vi "Begin.vi"(11 "Image Size":T1=enum."160x120") -> ()   [LabVIEW 2012]
doc: "Called before other user functions, this VI is expected to open initial I/O refnums, load in file data, and do all program initialization. Notice that the <B>error out</B> terminal is simply used for data flow. Wiring it to other structures or subVIs ensures that this VI runs first."
uses:
  <vilib>/Rock Robotics/WPI/Camera/WPI_CameraImageSize.ctl
  <vilib>/Rock Robotics/WPI/DriverStation/WPI_DriverStationRobotMode2.ctl
  <vilib>/Rock Robotics/WPI/Joystick/WPI_JoystickDeviceEnum.ctl
  <vilib>/Rock Robotics/WPI/CAN/Jaguar/SubVIs/WPI_CANJaguar_ControlMode.ctl
  <vilib>/Rock Robotics/WPI/CAN/Jaguar/SubVIs/WPI_CANJaguar_BrakeCoastMode.ctl
  <vilib>/Rock Robotics/WPI/CAN/Jaguar/SubVIs/WPI_CANJaguar_PositionReference.ctl
  Robot Global Data.vi
  <vilib>/Rock Robotics/WPI/MotorControl/WPI_MotorControlOpenCANJaguar.vi
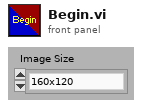
[diagram p1: front panel]
types:
  T1 = typedef "WPI_CameraImageSize.ctl" = enum16{"640x480", "320x240", "160x120"}
  T2 = typedef "WPI_CANJaguar_PositionReference.ctl" = u8
  T3 = typedef "WPI_CANJaguar_BrakeCoastMode.ctl" = enum8{"Jumper", "Brake", "Coast"}
  T4 = typedef "WPI_CANJaguar_ControlMode.ctl" = enum8{"Percent VBus", "Current", "Speed", "Position", "Voltage"}
  T5 = typedef "WPI_JoystickDeviceEnum.ctl" = enum16{"USB 1", "USB 2", "USB 3", "USB 4", "Kinect 1", "Kinect 2"}
  T6 = typedef "WPI_DriverStationRobotMode2.ctl" = enum16{"Autonomous Disabled", "Autonomous Enabled", "Teleop Disabled", "Teleop Enabled", "Timeout", "Finish", "Test Disabled", "Test Enabled"}
  T7 = typedef "WPI_JoystickDevRef.ctl" = cluster{"Device":T5}
  T8 = typedef "WPI_MotorControlDeviceRef.ctl" = cluster{"DeviceStatus":errorcluster, "Type":enum16{"PWM", "CAN"}, "PWM":cluster{"Digital Module":T9, "PWM Channel":T10, "DeadBand":T11}, "CAN":cluster{"Device Number":u8, "Control Mode":T4, "Semaphore":T12, "Max Vout":dbl}, "Invert":bool, "TransformRef":T13, "InvTransformRef":T13}
  T9 = typedef "FPGA_TypedefDigitalModule.ctl" = enum16{"Digital Module 1", "Digital Module 2"}
  T10 = typedef "FPGA_DIOPWMChannel.ctl" = enum8{"PWM 1", "PWM 2", "PWM 3", "PWM 4", "PWM 5", "PWM 6", "PWM 7", "PWM 8", "PWM 9", "PWM 10", "Invalid"}
  T11 = typedef "WPI_PWMDeadband.ctl" = cluster{"Name":string, "maxPositivePwm":i32, "minPositivePwm":i32, "centerPwm":i32, "maxNegativePwm":i32, "minNegativePwm":i32, "angularRange":u16}
  T12 = typedef "Semaphore RefNum" = refnum<k1>
  T13 = typedef "WPI_PWMTransform_ConPane.ctl" = refnum<vi>
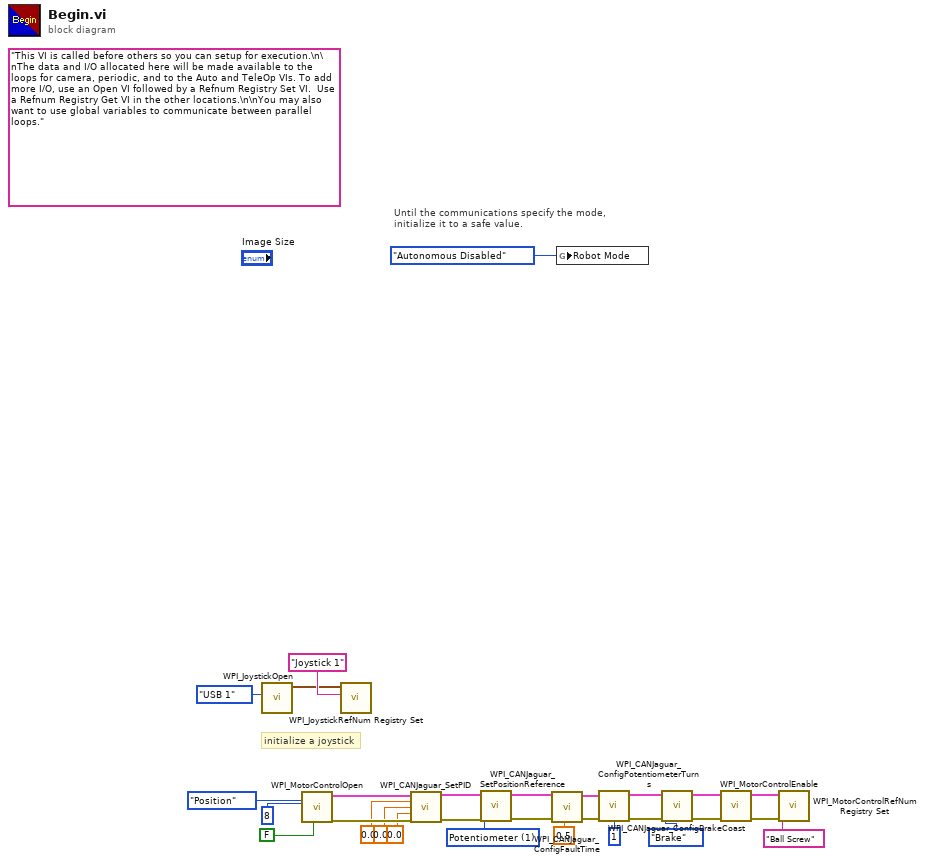
[diagram p0: block diagram]
diagram:
  w2 = T2 1 items=["Quad Encoder"=0, "Potentiometer"=1, "None"=255] ("Position Reference")
  (unwired) "This VI is called before others so you can setup for execution.\n\nThe data and I/O allocated here will be made available to the loops for camera, periodic, and to the Auto and TeleOp VIs. To add more I/O, use an Open VI followed by a Refnum Registry Set VI.  Use a Refnum Registry Get VI in the other locations.\n\nYou may also want to use global variables to communicate between parallel loops."
  # "initialize a joystick"
  # "Until the communications specify the mode,\ninitialize it to a safe value."
  n1 = call <vilib>:"WPI_JoystickOpen.vi"("JoystickDevice"=WPI_JoystickDeviceEnum."USB 1") -> ("JoystickDevRef"=w27:T7)  [unwired: 10 in]
  n2 = call-poly <vilib>:"WPI_MotorControlOpen.vi"("Invert"=FALSE, "Device Number"=u8 8, "Control Mode"=WPI_CANJaguar_ControlMode."Position") -> ("error out"=w19:errorcluster, "MotorControlDeviceRef"=w18:T8)  [unwired: 7 in]
  n3 = call <vilib>:"WPI_JoystickRefNum Registry Set.vi"("refnum name"="Joystick 1", "JoystickDevRef"=w27) -> ()  [unwired: 8 in, 2 out]
  n4 = call <vilib>:"WPI_CANJaguar_SetPID.vi"("CAN Jaguar Ref"=w18, "P"=0.0, "I"=0.0, "D"=0.0, "error in (no error)"=w19) -> ("CAN Jaguar Ref Out"=w25:T8, "error out"=w24:errorcluster)  [unwired: 9 in]
  n5 = call <vilib>:"WPI_CANJaguar_SetPositionReference.vi"("error in (no error)"=w24, "Position Reference"=w2, "CAN Jaguar Ref"=w25) -> ("error out"=w23:errorcluster, "CAN Jaguar Ref Out"=w22:T8)  [unwired: 7 in]
  n6 = call <vilib>:"WPI_CANJaguar_ConfigFaultTime.vi"("error in (no error)"=w23, "Fault Time (s)"=0.5, "CAN Jaguar Ref"=w22) -> ("error out"=w20:errorcluster, "CAN Jaguar Ref Out"=w21:T8)  [unwired: 7 in]
  n7 = global write "Robot Global Data.vi" "Robot Mode"(WPI_DriverStationRobotMode2."Autonomous Disabled" ("Robot Mode")) -> ()
  n8 = call <vilib>:"WPI_CANJaguar_ConfigPotentiometerTurns.vi"("error in (no error)"=w20, "Potentiometer Turns"=u16 1 ("Encoder Codes Per Rev"), "CAN Jaguar Ref"=w21) -> ("error out"=w14:errorcluster, "CAN Jaguar Ref Out"=w13:T8)  [unwired: 7 in]
  n9 = call <vilib>:"WPI_CANJaguar_ConfigBrakeCoast.vi"("error in (no error)"=w14, "Brake / Coast Mode"=WPI_CANJaguar_BrakeCoastMode."Brake", "CAN Jaguar Ref"=w13) -> ("error out"=w5:errorcluster, "CAN Jaguar Ref Out"=w6:T8)  [unwired: 7 in]
  n10 = call <vilib>:"WPI_MotorControlEnable.vi"("error in (no error)"=w5, "CAN Jaguar Ref"=w6) -> ("error out"=w3:errorcluster, "CAN Jaguar Ref Out"=w4:T8)  [unwired: 8 in]
  n11 = call <vilib>:"WPI_MotorControlRefNum Registry Set.vi"("error in (no error)"=w3, "refnum name"="Ball Screw", "MotorControlDevRef"=w4) -> ()  [unwired: 7 in, 2 out]
